vi "hReadChannels-UandP-2018.vi"(0 "FPGA VI Reference In":refnum<k20>, 2 "SampleTime":sgl=0.0004, 3 "final channel selection":i64[][](array[numeric]), 4 "kbolott_and_volume":sgl[][](array[numeric]), 5 "Nsamples":u32, 6 "tau_channels":sgl[](array[numeric]), 7 "error in":errorcluster, 8 "F_Ch":sgl[](array[numeric]), 9 "Scale(mV)":sgl[](array[numeric]), 10 "Offset (V)":dbl[](array[numeric]), 11 "av power array":refnum<vi>, 12 "single channel number":i64, 13 "single channel voltage":refnum<vi>, 14 "voltage array":refnum<vi>, 15 "tau_fact":sgl[](array[numeric]), 17 "current P_rad sample":refnum<vi>) -> (1 "Fehler":bool, 20 "FPGA VI Reference Out":refnum<k20>, 21 "PowerArray":sgl[][](array[numeric]), 25 "RawArray":sgl[][](array[numeric]), 27 "error out":errorcluster)   [LabVIEW 2014]
doc: "startet das einlesen und führt dies bis n Samples aus\nHier mit FIFO und IRQ."
uses:
  <vilib>/Utility/error.llb/Error Cluster From Error Code.vi
  <vilib>/rvi/errors/niLvFpgaAdjustHostInterfaceError.vi
  <vilib>/RVI Host/nirviSupport.llb/nirviErrorClusterFromErrorCode.vi
  <vilib>/rvi/interface/nirviReadWriteControl/nirviReadWriteControl.xnode
  FPGA Bitfiles/W7XBolo2017_FPGATarget_fmain2014_9xlV3GyHFfo.lvbitx
  f_main_2014.vi
  <vilib>/rvi/interface/nirviMethod/nirviMethod.xnode
  NiFpgaLv.dll
  <vilib>/rvi/interface/nirviMethod/StockFPGA_InlinedMethodWaitForMultipleIRQ.vi
  <vilib>/FPGAPlugInAG/PCI-7813R/niLvFpga_WaitOnIrq_PCI-7813R.vi
  <vilib>/FPGAPlugInAG/PCI-7813R/niLvFpga_AcknowledgeIrq_PCI-7813R.vi
  <vilib>/FPGAPlugInAG/PCI-7813R/niLvFpga_ReadFifo_PCI-7813R.vi
  <vilib>/rvi/errors/niLvFpgaMergeErrorWithErrorCode.vi
panel:
  out "single channel voltage":dbl
  in  "No. samples":i32=10
  in  "magic number":dbl=10.0
  out "single voltage array":dbl[](array[numeric])
  out "dU/dt":sgl[](array[numeric])
  out "U_0":dbl=5.0
  out "r_C":dbl=41.0
  out "omega":dbl
  out "av/f_OT*volume/k_bolo/V_cam":dbl
  out "average":dbl
  out "sum":dbl
  out "av/f_OT*volume/k_bolo":dbl
  out "average/f_OT":sgl
  out "av/f_OT*volume":dbl
  out "iterator":i32
  out "channel selected":i64
  out "volume element":sgl
  out "current power":sgl[](array[numeric])
  out "corrected voltage sample":sgl[](array[numeric])
  out "last U sample":sgl[](array[numeric])
  out "x*2^n":dbl[](array[numeric])
  out "av array":dbl[](array[numeric])
  out "V_Cam":dbl format="%#_13g"
  out "new level of override":i32
  out "rt prad average array":dbl[][](array[numeric])
  out "rawarray":sgl[][](array[numeric])
  out "powerarray":sgl[][](array[numeric])
  out "current sample array":sgl[](array[numeric])
  in  "wait ms":i32
  out "column":i32
  out "channel index":i32
  out "sample":i32
  out "current P_rad [MW]":dbl
  out "elec. channel selected":i64
  out "sate":string
  out "element of channel\nand sample":sgl
  out "channel number":i64
  out "Elements Remaining":u32
  out "STOP?":bool
  out "Timed Out":bool
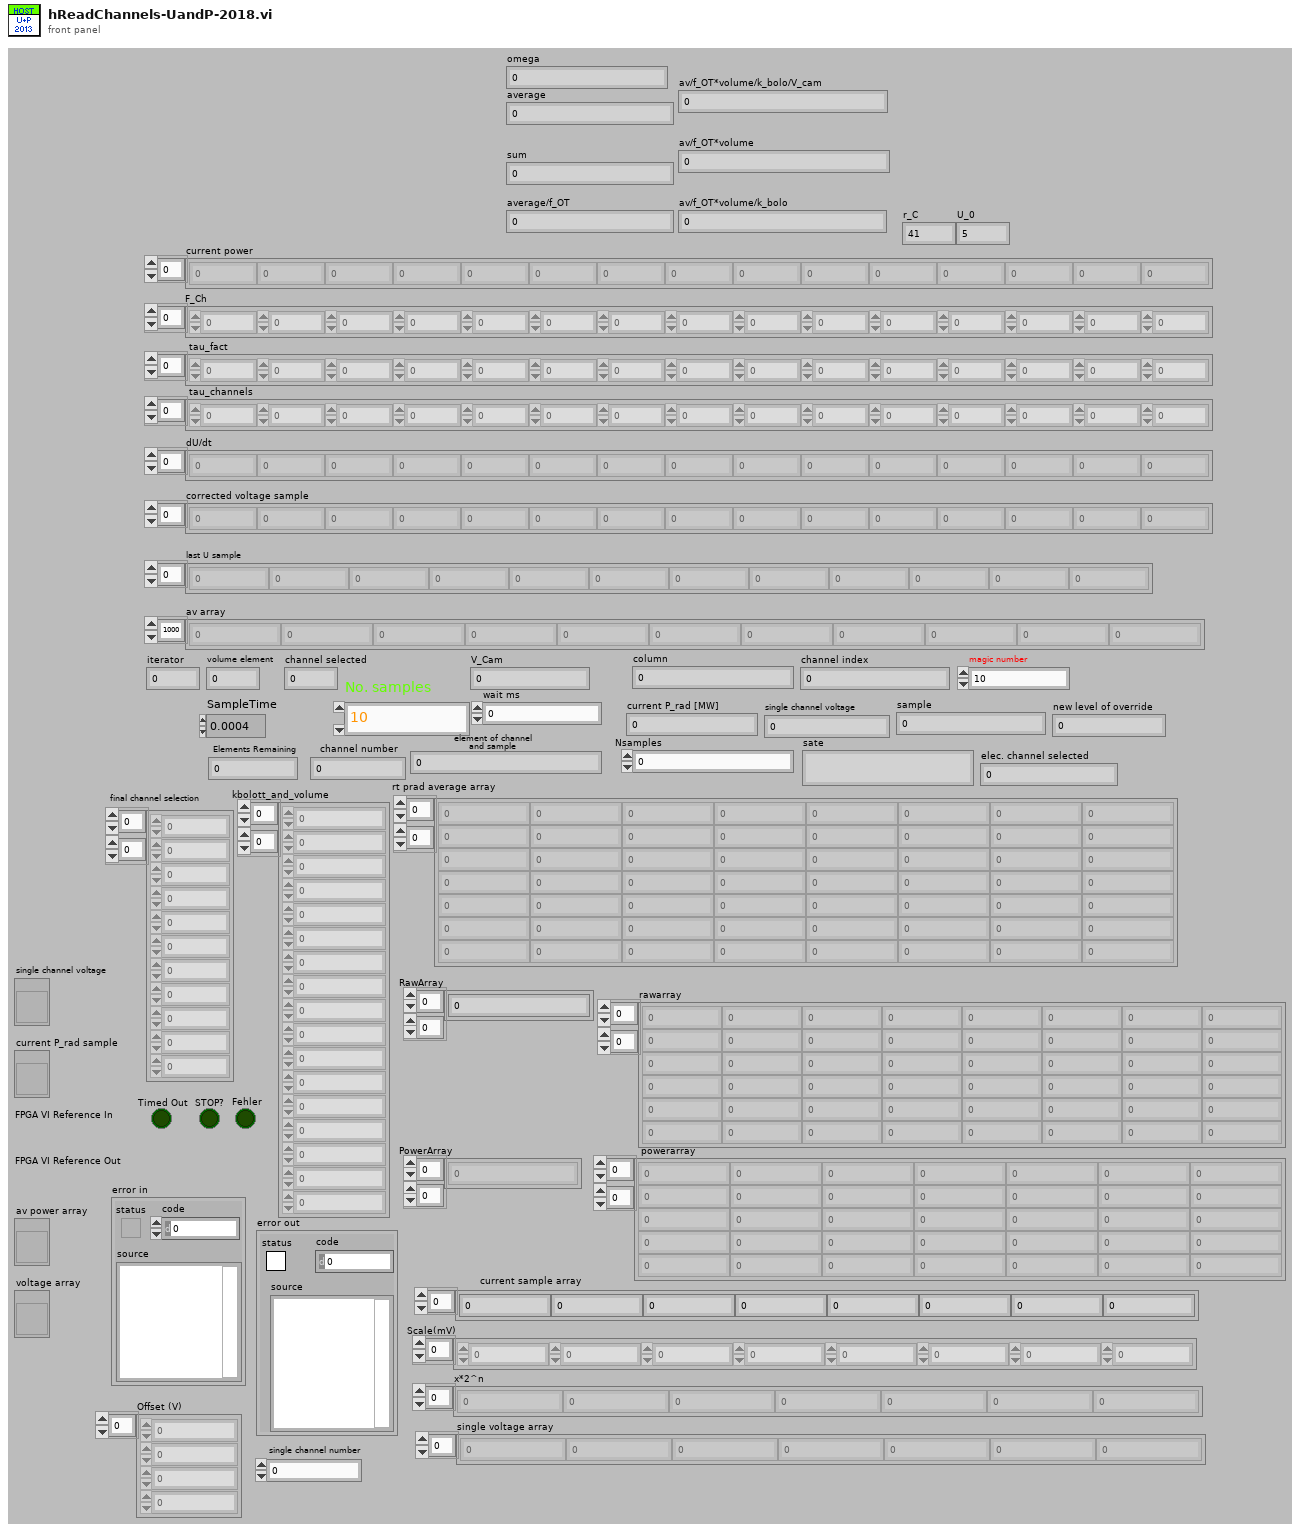
[diagram p1: front panel]
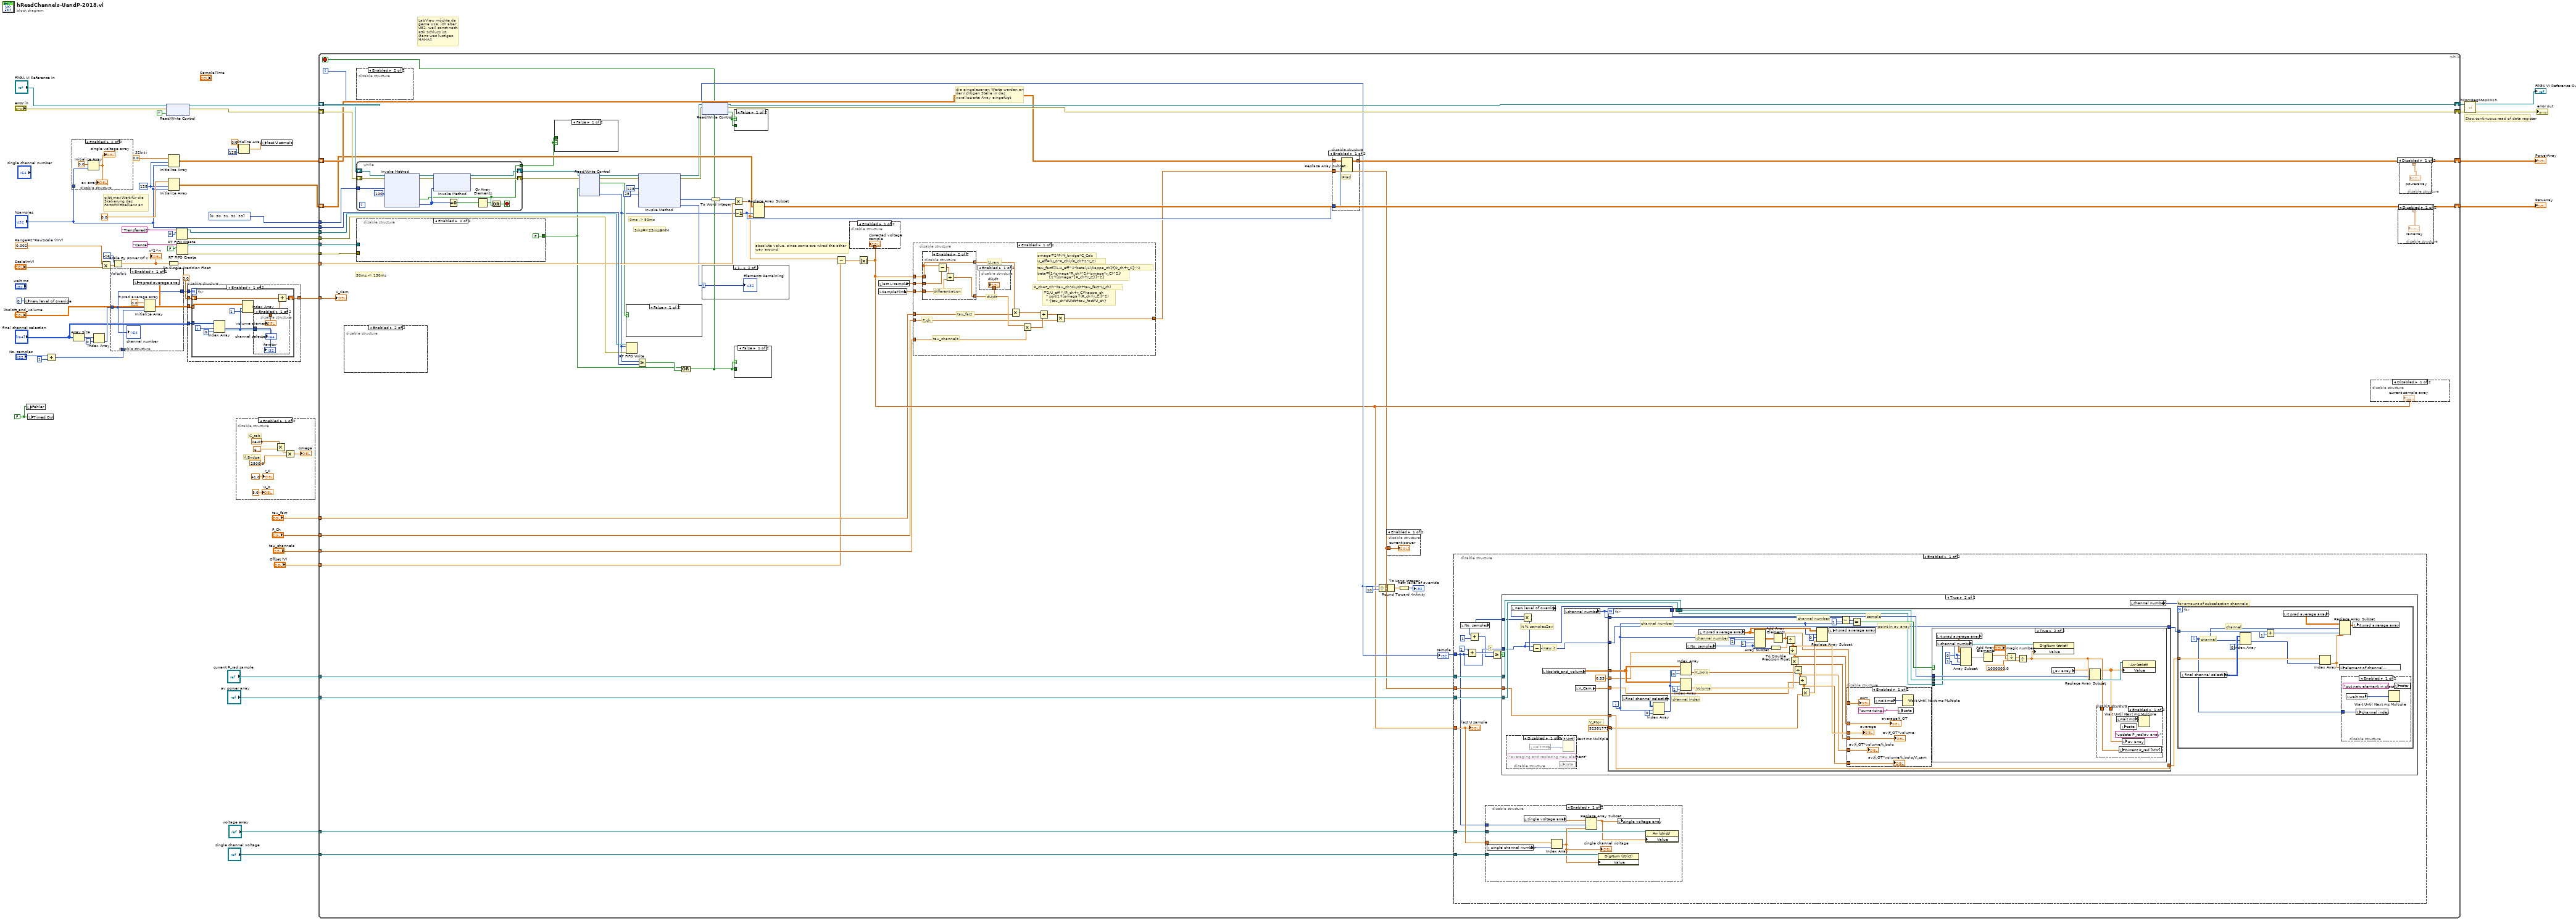
[diagram p0: block diagram]
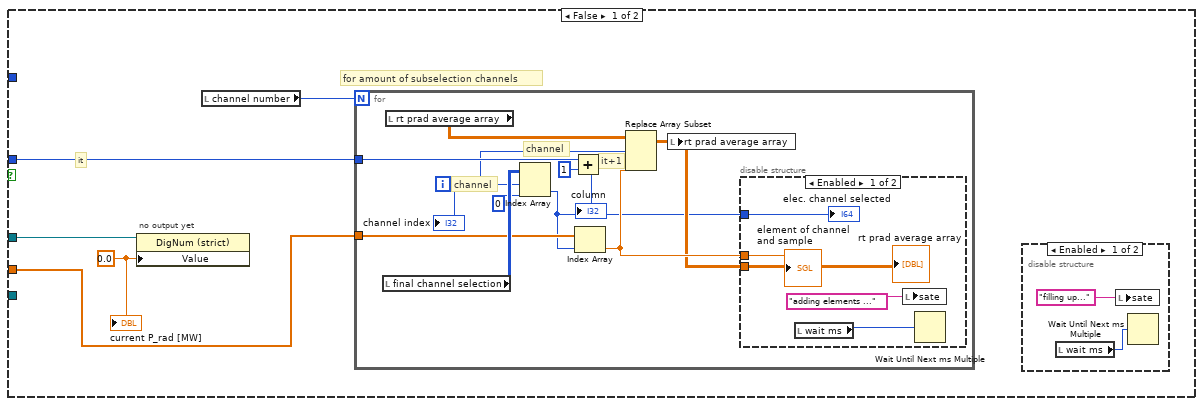
[diagram p9: hidden frame]
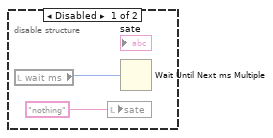
[diagram p18: hidden frame]
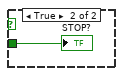
[diagram p19: hidden frame]
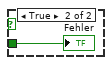
[diagram p20: hidden frame]
diagram:
  w29 = 0.002  # Range=2*RawScale (mV)
  w38 = 128 ("dimension size")
  w48 = sgl 0.0  # 32bit i
  w46 = FALSE
  # "Stop continuous read of data register"
  # "gibt maxWert für die Skalierung des Fortschrittbalkens an"
  # "LabView möchte da gerne U16, ich aber U32, weil sonst nach 65k Schluss ist. \nGanz was lustiges, HAHA!!"
  n1 = local write "new level of override"(i64 0 ("current level of override")) -> ()
  n2 = local write "Fehler"(w46) -> ()
  n3 = local write "Timed Out"(w46) -> ()
  n4 = Add(x="No. samples", y=1) -> (x+y=w1:i32)
  n5 = disable-structure shown="Enabled" {
    disable-tunnel: "Nsamples" -> [_ w59]
    frame Disabled {
    }
    frame Enabled {
      n6 = Initialize Array(0.0 ("element"), w59) -> (→"av array" →"single voltage array":dbl[])
    }
  }
  n7 = Array Size(array="final channel selection") -> (size(s)=w20:i32[])
  n8 = Index Array(array=w20, index=0) -> (element=w18:i32)
  n9 = Multiply(x=w29, y="Scale(mV)") -> (x*y=w30:dbl[])
  n10 = disable-structure shown="Enabled" {
    disable-tunnel: w18 -> [w61]
    disable-tunnel: [w61] -> w13
    disable-tunnel: w1 -> [w60]
    frame Enabled {
      n11 = Initialize Array "rt prad average array"(0.0 ("element"), w61, w60) -> (w62:dbl[][])
      n12 = local write "rt prad average array"(w62) -> ()
      "channel number" <- w61
    }
  }
  n13 = Scale By Power Of 2 "Volts/bit"(n=i16 -16, x=w30) -> (x*2^n=w31:dbl[])
  "x*2^n" <- w31
  n14 = xnode "Read/Write Control"("FPGA VI Reference In"="FPGA VI Reference In", "error in"="error in", "ADCRead"=TRUE) -> ("FPGA VI Reference Out"=w35:refnum<k20>, "error out"=w34:errorcluster)
  n15 = Initialize Array(w48, w38, "Nsamples") -> (w47:sgl[][])
  n16 = Initialize Array(sgl 0.0, w38, "Nsamples") -> (w56:sgl[][])
  n17 = To Single Precision Float(number=w31) -> (single precision float=w28:sgl[])
  n18 = RT FIFO Create(0:"Transferred1" ("name (unnamed)"), 1:u32 0) -> (8:w53:refnum<k33>, 11:w52:errorcluster)  [unwired: 2 in, 5 out]
  n19 = RT FIFO Create(0:"Cancel" ("name (unnamed)"), 1:FALSE) -> (8:w50:refnum<k33>, 11:w49:errorcluster)  [unwired: 2 in, 5 out]
  n20 = disable-structure shown="Enabled" {
    disable-tunnel: "kbolott_and_volume" -> [w68 _]
    disable-tunnel: "final channel selection" -> [w67 _]
    disable-tunnel: 0.0 -> [w66 _]
    disable-tunnel: [w65 _] -> w10
    disable-tunnel: w13 -> [w64 _]
    frame Enabled {
      n21 = for {
        N: w64 -> [_]
        tunnel: w68 -> [w77]
        tunnel: w67 -> [w75]
        shift-right: [w69] -> w65
        shift-left: w66 -> [w70]
        i -> [w76]
        n22 = Index Array(array=w75, index (row)=w76, index (col)=0 ("disabled index (col)")) -> (element=w72:i64)
        n23 = Index Array(array=w77, index (row)=w72, index (col)=1 ("disabled index (col)")) -> (element=w73:sgl)
        n24 = disable-structure shown="Enabled" {
          disable-tunnel: w76 -> [w80 _]
          disable-tunnel: w73 -> [w79 _]
          disable-tunnel: w72 -> [w78 _]
          frame Enabled {
            "volume element" <- w79
            "channel selected" <- w78
            "iterator" <- w80
          }
          frame Disabled {
          }
        }
        n25 = Add(x=w70, y=w73) -> (x+y=w69:dbl)
      }
    }
    frame Disabled {
    }
  }
  n26 = disable-structure shown="Enabled" {
    frame Enabled {
      # "C_cab"
      # "f_Bridge"
      n27 = Multiply(x=2e-09, y=6.283185307179586) -> (x*y=w85:dbl)
      n28 = Multiply(x=w85, y=2500.0) -> (x*y=→"omega":dbl)
      "r_C" <- 41.0
      "U_0" <- 5.0
    }
    frame Disabled {
    }
  }
  n29 = Initialize Array(sgl 0.0 ("element"), 128 ("dimension size")) -> (w15:sgl[])
  n30 = local write "last U sample"(w15) -> ()
  n31 = while {
    tunnel: "Nsamples" -> [w137]
    shift-right: [w127] -> w39
    shift-left: w56 -> [w131]
    shift-right: [w138] -> w45
    shift-left: w35 -> [w141]
    shift-right: [w139] -> w44
    shift-left: w34 -> [w140]
    tunnel: w53 -> [w136]
    tunnel: w52 -> [w135]
    tunnel: w50 -> [w134]
    tunnel: w49 -> [w133]
    shift-right: [w128] -> w40
    shift-left: w47 -> [w132]
    tunnel: w28 -> [w130]
    tunnel: i32[] [0, 30, 31, 32, 33] -> [w129]
    tunnel: "current P_rad sample" -> [w126]
    tunnel: "av power array" -> [w125]
    tunnel: w10 -> [w99]
    tunnel: "tau_fact" -> [w96]
    tunnel: "F_Ch" -> [w95]
    tunnel: "tau_channels" -> [w94]
    tunnel: "Offset (V)" -> [w90]
    tunnel: "single channel voltage" -> [w88]
    tunnel: "voltage array" -> [w89]
    i -> [w98]
    stop <- w124 stop-if-true
    # "absolute value, since some are wired the other\nway around"
    # "5ms=>25ms@MM"
    # "0ms -> 50ms"
    # "50ms -> 150ms"
    # "die eingelesenen Werte werden an der richtigen Stelle in das vorallozierte Array eingefügt"
    n32 = disable-structure shown="Enabled" {
      frame Disabled {
        n33 = local read "wait ms"() -> (w283:i32)
        n34 = local write "sate"("nothing") -> ()
        n35 = Wait Until Next ms Multiple(millisecond multiple=w283) -> ()  [unwired: 1 out]
      }
      frame Enabled {
      }
    }
    n36 = disable-structure shown="Enabled" {
      frame Disabled {
        n37 = call "Wait"("Count(uSec)"=u32 5) -> ()  [unwired: 1 out]
      }
      frame Enabled {
      }
    }
    n38 = while {
      tunnel: [w288] -> w110
      shift-right: [w290] -> w106
      shift-left: w141 -> [w297]
      shift-right: [w289] -> w107
      shift-left: w140 -> [w296]
      tunnel: w129 -> [w294]
      stop <- w287 stop-if-true
      n39 = xnode "Invoke Method"("FPGA VI Reference In"=w297, "error in"=w296, "IRQ Number(s)"=w294, "Timeout (ms)"=100) -> ("FPGA VI Reference Out"=w291:refnum<k20>, "error out"=w292:errorcluster, "Timed Out"=w288:bool, "IRQ(s) Asserted"=w293:i32[])
      n40 = xnode "Invoke Method"("FPGA VI Reference In"=w291, "error in"=w292, "IRQ Number(s)"=w293) -> ("FPGA VI Reference Out"=w290:refnum<k20>, "error out"=w289:errorcluster)
      n41 = Equal To 0?(x=w293) -> (x = 0?=w286:bool[])
      n42 = Or Array Elements(Boolean array=w286) -> (logical OR=w285:bool)
      n43 = Or(x=w285, y=w288) -> (x .or. y?=w287:bool)
    }
    n44 = disable-structure shown="Enabled" {
      disable-tunnel: [w303 FALSE] -> w122
      disable-tunnel: w134 -> [w302 _]
      disable-tunnel: w133 -> [w301 _]
      frame Disabled {
        # "Da es passieren kann, dass der letzte IRQ verschluckt wird, sichert dies der Timeoutwert von 50ms ab."
        n45 = RT FIFO Read(0:w302, 1:FALSE ("element"), 3:w301) -> (9:w303:bool)  [unwired: 5 out]
      }
      frame Enabled {
      }
    }
    n46 = case shown="False" w110 {
      tunnel: w110 -> [_ w311]
      frame False {
      }
      frame True {
        "Timed Out" <- w311
      }
    }
    n47 = xnode "Read/Write Control"("FPGA VI Reference In"=w106, "error in"=w107, "cancel"=w122) -> ("FPGA VI Reference Out"=w120:refnum<k20>, "error out"=w119:errorcluster, "Timeout"=w121:bool, "ScanID"=w117:u32)
    n48 = case shown="False" w121 {
      selector: w121 -> [_ w337]
      frame False {
      }
      frame True {
        n49 = local write "Fehler"(w337) -> ()
      }
    }
    n50 = RT FIFO Write(0:w136, 1:w117, 3:w135) -> ()  [unwired: 1 in, 5 out]
    n51 = Greater Or Equal?(x=w117, y=w137) -> (x >= y?=w123:bool)
    n52 = xnode ("Invoke Method")("FPGA VI Reference In"=w120, "error in"=w119, "Number of Elements"=u32 128, "Timeout (ms)"=25 ("Timeout")) -> ("FPGA VI Reference Out"=w112:refnum<k20>, "error out"=w111:errorcluster, "Data"=w114:u32[], "Elements Remaining"=w109:u32)
    n53 = Compound Arithmetic op=OR(w122, w123) -> (w124:bool)
    n54 = xnode "Read/Write Control"("FPGA VI Reference In"=w112, "error in"=w111) -> ("FPGA VI Reference Out"=w138:refnum<k20>, "error out"=w139:errorcluster, "Fifo-Fehler"=w108:bool)
    n55 = case shown="1.." w109 {
      selector: w109 -> [_ w310]
      frame 0, Default {
      }
      frame 1.. {
        "Elements Remaining" <- w310
      }
    }
    n56 = To Word Integer(number=w114) -> (16bit integer=w113:i16[])
    n57 = Multiply(x=w113, y=w130) -> (x*y=w91:sgl[])
    n58 = Decrement(x=w117) -> (x-1=w118:u32)
    n59 = case shown="False" w108 {
      tunnel: w108 -> [_ w299]
      frame False {
      }
      frame True {
        "Fehler" <- w299
      }
    }
    n60 = case shown="False" w124 {
      tunnel: w124 -> [_ w298]
      frame False {
      }
      frame True {
        "STOP?" <- w298
      }
    }
    n61 = Replace Array Subset(array=w131, new element=w91, index (col)=w118) -> (w127:sgl[][])  [unwired: 1 in]
    n62 = Subtract(x=w91, y=w90) -> (x-y=w92:dbl[])
    n63 = Absolute Value(x=w92) -> (abs(x)=w97:dbl[])
    n64 = disable-structure shown="Enabled" {
      disable-tunnel: w97 -> [w143 _]
      frame Enabled {
        "corrected voltage sample" <- w143
      }
      frame Disabled {
      }
    }
    n65 = local read "last U sample"() -> (w101:sgl[])
    n66 = local read "SampleTime"() -> (w100:sgl)
    n67 = disable-structure shown="Enabled" {
      disable-tunnel: w97 -> [w323 w335]
      disable-tunnel: w101 -> [w322 _]
      disable-tunnel: w100 -> [w321 _]
      disable-tunnel: w96 -> [w315 _]
      disable-tunnel: w95 -> [w313 _]
      disable-tunnel: w94 -> [w318 _]
      disable-tunnel: [w312 w335] -> w93
      frame Enabled {
        # "beta=[1-(omega*R_ch)^2+(omega*r_C)^2]/\n         {1+[omega*{R_ch+r_C}]^2}"
        # "tau_fact[((1-U_eff^2*beta)/4)/kappa_ch]/{R_ch+r_C}^2"
        # "U_eff=(U_0*R_Ch)/(R_ch+2*r_C)"
        # "omega=2*Pi*f_bridge*C_Cab"
        # "=2/U_eff * (R_ch+r_C)*kappa_ch\n  * sqrt(1+[omega+(R_ch+r_C)]^2)\n  * {tau_ch*dU/dt+tau_fact*U_ch}"
        # "P_ch=F_Ch*(tau_ch*dU/dt+tau_fact*U_ch)"
        # "tau_channels"
        # "F_ch"
        # "tau_fact"
        # "U_raw"
        # "dU/dt"
        n68 = disable-structure shown="Enabled" {
          disable-tunnel: w323 -> [w329 w334]
          disable-tunnel: [w328 w330] -> w319
          disable-tunnel: [w325 w334] -> w320
          disable-tunnel: w322 -> [_ w333]
          disable-tunnel: w321 -> [_ w331]
          frame Disabled {
            n69 = call "Savitzky Golay Filter PtByPt with Derivative861.vi"("order polynomial"=2, "side points"=31, "x"=w329) -> ("Filtered Derivative"=w328:dbl[], "Filtered x"=w325:dbl[])  [unwired: 1 in, 6 out]
          }
          frame Enabled {
            # "differentiation"
            n70 = Subtract(x=w334, y=w333) -> (x-y=w332:dbl[])
            n71 = Divide(x=w332, y=w331) -> (x/y=w330:dbl[])
          }
        }
        n72 = disable-structure shown="Enabled" {
          disable-tunnel: w319 -> [w324 _]
          frame Enabled {
            "dU/dt" <- w324
          }
          frame Disabled {
          }
        }
        n73 = Multiply(x=w320, y=w315) -> (x*y=w314:dbl[])
        n74 = Multiply(x=w319, y=w318) -> (x*y=w317:dbl[])
        n75 = Add(x=w314, y=w317) -> (x+y=w316:dbl[])
        n76 = Multiply(x=w316, y=w313) -> (x*y=w312:dbl[])
      }
      frame Disabled {
      }
    }
    n77 = disable-structure shown="Enabled" {
      disable-tunnel: w132 -> [w308 w309]
      disable-tunnel: [w307 w309] -> w128
      disable-tunnel: w118 -> [w305 _]
      disable-tunnel: w93 -> [w306 _]
      frame Enabled {
        # "Prad"
        n78 = Replace Array Subset(array=w308, new element=w306, index (col)=w305) -> (w307:sgl[][])  [unwired: 1 in]
      }
      frame Disabled {
      }
    }
    n79 = Divide(x=w98, y=10) -> (x/y=w104:dbl)
    n80 = Round Toward -Infinity(1:w104) -> (0:w103:dbl)
    n81 = disable-structure shown="Enabled" {
      disable-tunnel: w93 -> [w142 _]
      frame Enabled {
        "current power" <- w142
      }
      frame Disabled {
      }
    }
    n82 = To Long Integer(number=w103) -> (32bit integer=→"new level of override":i32)
    n83 = disable-structure shown="Enabled" {
      disable-tunnel: w98 -> [w148 _]
      disable-tunnel: w126 -> [w153 _]
      disable-tunnel: w125 -> [w152 _]
      disable-tunnel: w93 -> [w151 _]
      disable-tunnel: w97 -> [w150 _]
      disable-tunnel: w89 -> [w147 _]
      disable-tunnel: w88 -> [w149 _]
      frame Enabled {
        # "it"
        n84 = local read "No. samples"() -> (w144:i32)
        n85 = Add(x=1, y=w148) -> (x+y=w154:i32)
        n86 = Add(x=w144, y=i64 1) -> (x+y=w145:i64)
        n87 = disable-structure shown="Enabled" {
          disable-tunnel: w150 -> [w164 _]
          disable-tunnel: w149 -> [w162 _]
          disable-tunnel: w148 -> [w160 _]
          disable-tunnel: w147 -> [w158 _]
          frame Enabled {
            n88 = local read "single channel number"() -> (w163:i64)
            n89 = local read "single voltage array"() -> (w161:dbl[])
            n90 = Index Array(array=w164, index=w163) -> (element=w159:dbl)
            "single channel voltage" <- w159
            n91 = Replace Array Subset(array=w161, new element=w159, index=w160) -> (w157:dbl[])
            n92 = property class="DigNum (strict)"(reference=w162, "Value"=w159) -> ()  [unwired: 1 in, 2 out]
            n93 = local write "single voltage array"(w157) -> ()
            n94 = property class="Arr (strict)"(reference=w158, "Value"=w157) -> ()  [unwired: 1 in, 2 out]
          }
          frame Disabled {
          }
        }
        n95 = Greater Or Equal?(x=w154, y=w145) -> (x >= y?=w156:bool)
        n96 = case shown="True" w156 {
          tunnel: w148 -> [w165 w189]
          tunnel: w153 -> [w168 w191]
          tunnel: w152 -> [_ w192]
          tunnel: w151 -> [w166 w190]
          tunnel: w144 -> [_ w188]
          frame False {
            w167 = 0.0 ("Value")
            # "it"
            # "for amount of subselection channels"
            # "no output yet"
            n97 = property class="DigNum (strict)"(reference=w168, "Value"=w167) -> ()  [unwired: 1 in, 2 out]
            n98 = local read "channel number"() -> (w169:i64)
            n99 = for {
              N: w169 -> [_]
              tunnel: w165 -> [w178]
              tunnel: w166 -> [w176]
              i -> [w173]
              # "channel"
              # "channel"
              # "it+1"
              n100 = local read "final channel selection"() -> (w182:i64[][])
              n101 = local read "rt prad average array"() -> (w177:dbl[][])
              n102 = Index Array(array=w182, index (row)=w173, index (col)=0 ("disabled index (col)")) -> (element=w172:i64)
              n103 = Add(x=w178, y=1) -> (x+y=w179:i32)
              "column" <- w179
              n104 = Index Array(array=w176, index=w172) -> (element=w175:dbl)
              n105 = Replace Array Subset(array=w177, new element=w175, index (row)=w173, index (col)=w179) -> (w174:dbl[][])
              n106 = local write "rt prad average array"(w174) -> ()
              n107 = disable-structure shown="Enabled" {
                disable-tunnel: w172 -> [w186 _]
                disable-tunnel: w175 -> [w184 _]
                disable-tunnel: w174 -> [w183 _]
                frame Enabled {
                  n108 = local read "wait ms"() -> (w185:i32)
                  n109 = local write "sate"("adding elements ...") -> ()
                  n110 = Wait Until Next ms Multiple(millisecond multiple=w185) -> ()  [unwired: 1 out]
                  "element of channel\nand sample" <- w184
                  "elec. channel selected" <- w186
                  "rt prad average array" <- w183
                }
                frame Disabled {
                }
              }
              "channel index" <- w173
            }
            n111 = disable-structure shown="Enabled" {
              frame Enabled {
                n112 = local read "wait ms"() -> (w170:i32)
                n113 = local write "sate"("filling up...") -> ()
                n114 = Wait Until Next ms Multiple(millisecond multiple=w170) -> ()  [unwired: 1 out]
              }
              frame Disabled {
              }
            }
            "current P_rad [MW]" <- w167
          }
          frame True {
            # "V_Ptor"
            # "new it"
            # "it % samples2av"
            # "for amount of subselection channels"
            n115 = disable-structure shown="Disabled" {
              frame Disabled {
                n116 = local read "wait ms"() -> (w204:i32)
                n117 = local write "sate"("averaging and replacing new element") -> ()
                n118 = Wait Until Next ms Multiple(millisecond multiple=w204) -> ()  [unwired: 1 out]
              }
              frame Enabled {
              }
            }
            n119 = local read "new level of override"() -> (w202:i32)
            n120 = Multiply(x=w202, y=w188) -> (x*y=w201:i32)
            n121 = Subtract(x=w189, y=w201) -> (x-y=w199:i32)
            n122 = local read "kbolott_and_volume"() -> (w200:sgl[][])
            n123 = local read "channel number"() -> (w194:i64)
            n124 = local read "V_Cam"() -> (w196:dbl)
            n125 = for {
              N: w194 -> [_]
              tunnel: w200 -> [w236]
              tunnel: [w241] -> w195
              tunnel: w190 -> [w241]
              tunnel: [w221] -> w193
              tunnel: w199 -> [w221]
              tunnel: 52381772.0 -> [w215]
              tunnel: 0.53 -> [w219]
              tunnel: w196 -> [w216]
              tunnel: w194 -> [w222]
              tunnel: w189 -> [w227]
              tunnel: w192 -> [w226]
              tunnel: w191 -> [w223]
              i -> [w220]
              # "channel number"
              # "channel number"
              # "point in av array"
              # "sample"
              # "channel number"
              # "K_bolo"
              # "Volume"
              # "channel index"
              n126 = local read "final channel selection"() -> (w240:i64[][])
              n127 = Index Array(array=w240, index (row)=w220, index (col)=0 ("disabled index (col)")) -> (element=w237:i64)
              n128 = Index Array(array=w236, index (row)=w237, index (col)=0 ("disabled index (col)")) -> (element=w217:sgl)
              n129 = Index Array(array=w236, index (row)=w237, index (col)=1 ("disabled index (col)")) -> (element=w218:sgl)
              n130 = local read "No. samples"() -> (w207:i32)
              n131 = local read "rt prad average array"() -> (w231:dbl[][])
              n132 = Array Subset(array=w231, index (row)=w220, length (row)=1, index (col)=1 ("index"), length (col)=w207) -> (w232:dbl[][])
              n133 = To Double Precision Float(number=w207) -> (double precision float=w206:dbl)
              n134 = Add Array Elements(numeric array=w232) -> (sum=w212:dbl)
              n135 = Divide(x=w212, y=w206) -> (x/y=w213:dbl)
              n136 = Divide(x=w213, y=w219) -> (x/y=w211:dbl)
              n137 = Multiply(x=w211, y=w218) -> (x*y=w210:dbl)
              n138 = Divide(x=w210, y=w217) -> (x/y=w209:dbl)
              n139 = Divide(x=w209, y=w216) -> (x/y=w208:dbl)
              n140 = Multiply(x=w208, y=w215) -> (x*y=w214:dbl)
              n141 = Replace Array Subset(array=w231, new element=w214, index (row)=w220, index (col)=0 ("disabled index (col)")) -> (w229:dbl[][])
              n142 = local write "rt prad average array"(w229) -> ()
              n143 = Subtract(x=w222, y=i64 1) -> (x-y=w225:i64)
              n144 = disable-structure shown="Enabled" {
                disable-tunnel: w213 -> [w247 _]
                disable-tunnel: w212 -> [w246 _]
                disable-tunnel: w211 -> [w245 _]
                disable-tunnel: w210 -> [w244 _]
                disable-tunnel: w209 -> [w243 _]
                disable-tunnel: w208 -> [w242 _]
                frame Enabled {
                  n145 = local read "wait ms"() -> (w249:i32)
                  n146 = local write "sate"("sumarizing...") -> ()
                  n147 = Wait Until Next ms Multiple(millisecond multiple=w249) -> ()  [unwired: 1 out]
                  "av/f_OT*volume/k_bolo" <- w243
                  "average/f_OT" <- w245
                  "av/f_OT*volume" <- w244
                  "sum" <- w246
                  "average" <- w247
                  "av/f_OT*volume/k_bolo/V_cam" <- w242
                }
                frame Disabled {
                }
              }
              n148 = Equal?(x=w225, y=w220) -> (x = y?=w228:bool)
              n149 = case shown="True" w228 {
                tunnel: w227 -> [_ w260]
                tunnel: w226 -> [_ w259]
                tunnel: w223 -> [_ w258]
                frame False {
                }
                frame True {
                  w253 = 0 ("index")
                  n150 = local read "rt prad average array"() -> (w262:dbl[][])
                  n151 = local read "channel number"() -> (w254:i64)
                  n152 = Array Subset(array=w262, index (row)=w253, length (row)=w254, index (col)=w253, length (col)=1 ("index")) -> (w264:dbl[][])
                  n153 = Add Array Elements(numeric array=w264) -> (sum=w251:dbl)
                  n154 = Divide(x=w251, y="magic number") -> (x/y=w252:dbl)
                  n155 = Divide(x=w252, y=1000000.0) -> (x/y=w256:dbl)
                  n156 = property class="DigNum (strict)"(reference=w258, "Value"=w256) -> ()  [unwired: 1 in, 2 out]
                  n157 = local read "av array"() -> (w261:dbl[])
                  n158 = Replace Array Subset(array=w261, new element=w256, index=w260) -> (w255:dbl[])
                  n159 = disable-structure shown="Enabled" {
                    disable-tunnel: w256 -> [w266 _]
                    disable-tunnel: w255 -> [w265 _]
                    frame Enabled {
                      n160 = local read "wait ms"() -> (w268:i32)
                      n161 = local write "current P_rad [MW]"(w266) -> ()
                      n162 = local write "sate"("update P_rad/av array") -> ()
                      n163 = local write "av array"(w265) -> ()
                      n164 = Wait Until Next ms Multiple(millisecond multiple=w268) -> ()  [unwired: 1 out]
                    }
                    frame Disabled {
                    }
                  }
                  n165 = property class="Arr (strict)"(reference=w259, "Value"=w255) -> ()  [unwired: 1 in, 2 out]
                }
              }
            }
            n166 = local read "channel number"() -> (w203:i64)
            n167 = for {
              N: w203 -> [_]
              tunnel: w193 -> [w275]
              tunnel: w195 -> [w273]
              i -> [w271]
              # "channel"
              # "channel"
              n168 = local read "final channel selection"() -> (w279:i64[][])
              n169 = Index Array(array=w279, index (row)=w271, index (col)=0 ("disabled index (col)")) -> (element=w269:i64)
              n170 = Add(x=w275, y=1) -> (x+y=w276:i32)
              n171 = local read "rt prad average array"() -> (w274:dbl[][])
              n172 = Index Array(array=w273, index=w269) -> (element=w270:dbl)
              n173 = local write "element of channel\nand sample"(w270) -> ()
              n174 = Replace Array Subset(array=w274, new element=w270, index (row)=w271, index (col)=w276) -> (w272:dbl[][])
              n175 = disable-structure shown="Enabled" {
                disable-tunnel: w271 -> [w280 _]
                frame Enabled {
                  n176 = local read "wait ms"() -> (w281:i32)
                  n177 = local write "channel index"(w280) -> ()
                  n178 = Wait Until Next ms Multiple(millisecond multiple=w281) -> ()  [unwired: 1 out]
                  n179 = local write "sate"("put new element in place") -> ()
                }
                frame Disabled {
                }
              }
              n180 = local write "rt prad average array"(w272) -> ()
            }
          }
        }
        "last U sample" <- w150
      }
      frame Disabled {
      }
    }
    n181 = disable-structure shown="Disabled" {
      disable-tunnel: w97 -> [w340 _]
      frame Disabled {
        "current sample array" <- w340
      }
      frame Enabled {
      }
    }
    n182 = disable-structure shown="Disabled" {
      disable-tunnel: w127 -> [w338 _]
      frame Disabled {
        "rawarray" <- w338
      }
      frame Enabled {
      }
    }
    n183 = disable-structure shown="Disabled" {
      disable-tunnel: w128 -> [w339 _]
      frame Disabled {
        "powerarray" <- w339
      }
      frame Enabled {
      }
    }
    "sample" <- w98
    "V_Cam" <- w99
  }
  "RawArray" <- w39
  "PowerArray" <- w40
  n184 = call "hComRegStop2013.vi"("error in"=w44, "FPGA VI Reference In"=w45) -> ("error out"=→"error out":errorcluster, "FPGA VI Reference Out"=→"FPGA VI Reference Out":refnum<k20>)  [unwired: 3 in, 1 out]
